vi "subvimotor.vi"(7 "PWM Ref Out":T1, 8 "error in (no error)":errorcluster, 9 "freq [Hz] 3":dbl, 10 "null offset 3":bool, 11 "position [%FS] 3":dbl) -> (1 "Numeric":dbl, 2 "Numeric 2":dbl, 3 "position [%FS]":dbl)   [LabVIEW 2017]
uses:
  <vilib>/myRIO/Instrument Drivers/Onboard IO/PWM/typedefs/PWM Reference.ctl
  <vilib>/myRIO/Common/Instrument Driver Framework/Utilities/typedefs/myRIO Generic Hardware Reference.ctl
  <vilib>/myRIO/Common/Instrument Driver Framework/Utilities/typedefs/Hardware Version Enum.ctl
  <vilib>/myRIO/Common/Instrument Driver Framework/Utilities/typedefs/myRIO v1.0 Reference.ctl
  <vilib>/myRIO/Common/Instrument Driver Framework/Utilities/typedefs/Generic FPGA Reference.ctl
  <vilib>/myRIO/Common/Instrument Driver Framework/myRIO v1.0/PWM/typedefs/PWM Channels Enum.ctl
  <vilib>/myRIO/Instrument Drivers/Onboard IO/PWM/typedefs/PWM Configuration.ctl
  <vilib>/Utility/error.llb/Error Cluster From Error Code.vi
  <vilib>/myRIO/Common/Instrument Driver Framework/myRIO v1.0/PWM/vis/myRIO v1.0 Write PWM.vi
  <vilib>/myRIO/Instrument Drivers/Onboard IO/PWM/PWM.lvlib
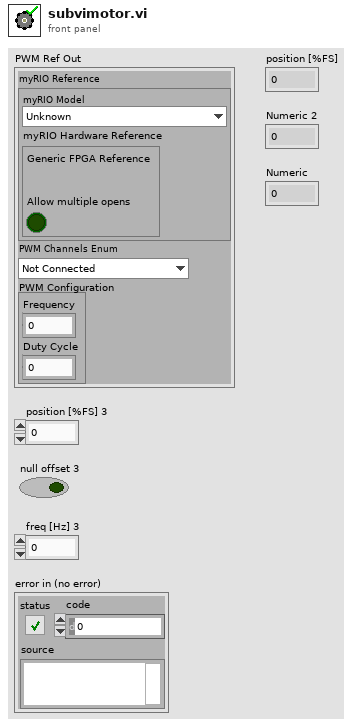
[diagram p1: front panel]
types:
  T1 = typedef "PWM.lvlib/PWM Reference.ctl" = cluster{"myRIO Reference":T2, "PWM Channels Enum":T6, "PWM Configuration":T7}
  T2 = typedef "myRIO Generic Hardware Reference.ctl" = cluster{"myRIO Model":T3, "myRIO Hardware Reference":T4}
  T3 = typedef "Hardware Version Enum.ctl" = enum16{"Unknown", "myRIO-1900", "myRIO-1950", "roboRIO", "NI ELVIS RIO CM"}
  T4 = typedef "myRIO v1.0 Reference.ctl" = cluster{"Generic FPGA Reference":T5, "Allow multiple opens":bool}
  T5 = typedef "Generic FPGA Reference.ctl" = refnum<k20>
  T6 = typedef "PWM Channels Enum.ctl" = enum16{"Not Connected", "C/PWM0", "C/PWM1", "A/PWM0", "A/PWM1", "A/PWM2", "B/PWM0", "B/PWM1", "B/PWM2", "PWM/PWM0", "PWM/PWM1", "PWM/PWM2", "PWM/PWM3", "PWM/PWM4", "PWM/PWM5", "PWM/PWM6", "PWM/PWM7", "PWM/PWM8", "PWM/PWM9"}
  T7 = typedef "PWM.lvlib/PWM Configuration.ctl" = cluster{"Frequency":dbl, "Duty Cycle":dbl}
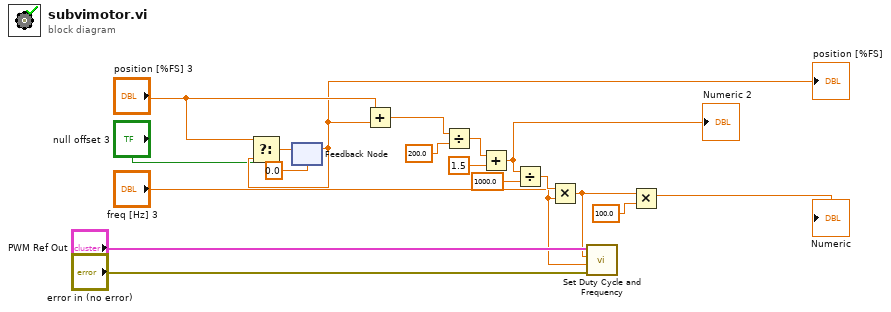
[diagram p0: block diagram]
diagram:
  n1 = feedback #1(0.0 ("position [%FS]")) -> (w10:dbl)
  "position [%FS]" <- w10
  n2 = Select(t="position [%FS] 3", s="null offset 3", f=w10) -> (s? t:f=w8:dbl)
  n3 = feedback-in #1(w8) -> ()
  n4 = Add(x="position [%FS] 3", y=w10) -> (x+y=w9:dbl)
  n5 = Divide(x=w9, y=200.0) -> (x/y=w2:dbl)
  n6 = Add(x=w2, y=1.5) -> (x+y=w4:dbl)
  "Numeric 2" <- w4
  n7 = Divide(x=w4, y=1000.0) -> (x/y=w12:dbl)
  n8 = Multiply(x=w12, y="freq [Hz] 3") -> (x*y=w15:dbl)
  n9 = call <vilib>:"Set Duty Cycle and Frequency.vi"("error in (no error)"="error in (no error)", "Frequency [Hz]"="freq [Hz] 3", "Duty Cycle"=w15, "PWM Ref In"="PWM Ref Out") -> ()  [unwired: 5 in, 2 out]
  n10 = Multiply(x=w15, y=100.0) -> (x*y=→"Numeric":dbl)
